vi "check RTU validity.vi"(8 "error in (no error)":errorcluster, 10 "unit ID":u8, 11 "unsigned byte array":u8[](array[numeric])) -> (0 "error out":errorcluster, 1 "valid packet":bool, 2 "valid PDU":bool, 3 "Modbus Data Unit out":refnum<class "Modbus Data Unit.lvclass">)   [LabVIEW 2012, in "RTU Data Unit.lvclass"]
uses:
  RTU Data Unit.lvclass
  Modbus Data Unit/Modbus Data Unit.lvclass
  Modbus Data Unit/Modbus Data Unit.lvclass/Modbus Data Unit.ctl
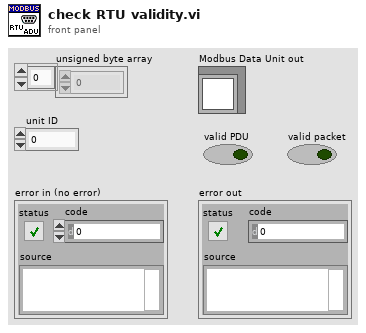
[diagram p1: front panel]
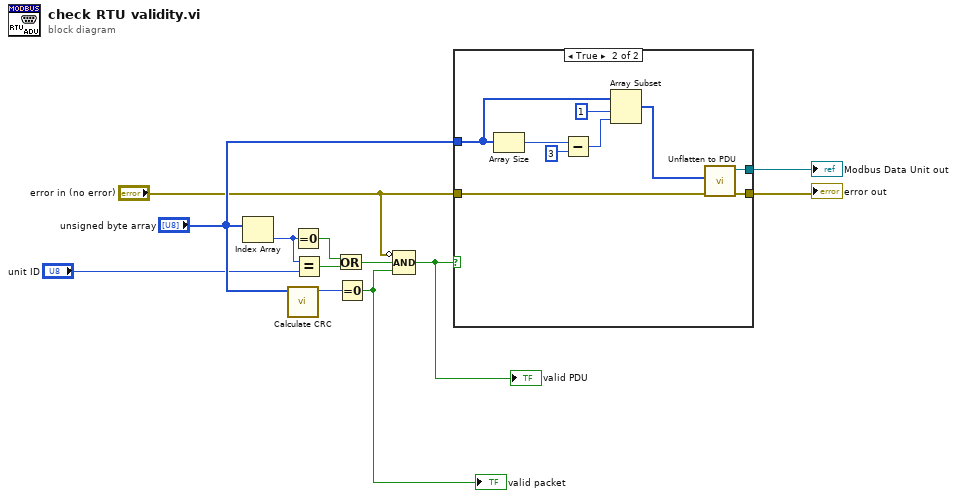
[diagram p0: block diagram]
diagram:
  n1 = Index Array(array="unsigned byte array") -> (element=w4:u8)  [unwired: 1 in]
  n2 = call "Calculate CRC.vi"("data"="unsigned byte array") -> ("CRC-16"=w3:u16)  [unwired: 10 in]
  n3 = Equal To 0?(x=w4) -> (x = 0?=w5:bool)
  n4 = Equal?(x=w4, y="unit ID") -> (x = y?=w6:bool)
  n5 = Or(x=w5, y=w6) -> (x .or. y?=w8:bool)
  n6 = Equal To 0?(x=w3) -> (x = 0?=w2:bool)
  "valid packet" <- w2
  n7 = Compound Arithmetic op=AND(invert "error in (no error)", w8, w2) -> (w1:bool)
  "valid PDU" <- w1
  n8 = case shown="True" w1 {
    tunnel: "error in (no error)" -> [w13 w17]
    tunnel: "unsigned byte array" -> [_ w16]
    tunnel: [w13 w15] -> w11
    tunnel: [_ w14] -> w12
    frame False {
    }
    frame True {
      n9 = Array Size(array=w16) -> (size(s)=w20:i32)
      n10 = Subtract(x=w20, y=3) -> (x-y=w18:i32)
      n11 = Array Subset(array=w16, index=1, length=w18) -> (w22:u8[])
      n12 = call "Unflatten to PDU.vi"("error in"=w17, "modbus data unit data"=w22) -> ("error out"=w15:errorcluster, "modbus data unit out"=w14:refnum<class "Modbus Data Unit.lvclass">)  [unwired: 8 in]
    }
  }
  "Modbus Data Unit out" <- w12
  "error out" <- w11
